vi "ReadSetPoint Example.vi"() -> ()   [LabVIEW 2019]
uses:
  BrooksDLL.dll
panel:
  out "Unit Comment (if Pressure)":string
  out "Unit Comment (if Flow)":string
  out "Unit Code":u8
  out "Set Point Value":sgl format="%.2f"
  out "S2 String":string
  out "S1 String":string
  out "S2":u8 format="%.0x"
  out "S1":u8 format="%.0x"
  out "Function Output Comment":string
  out "SetPoint %":sgl format="%.2f"
  out "output param":i32
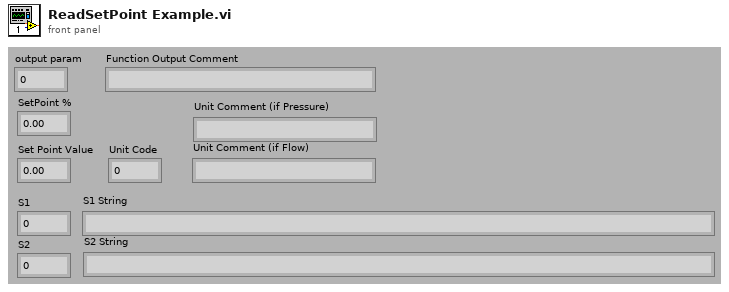
[diagram p1: front panel]
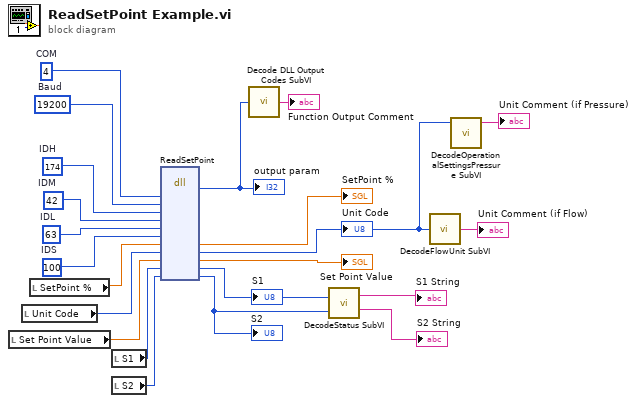
[diagram p0: block diagram]
diagram:
  w17 = u8 100  # IDS
  w18 = u8 63  # IDL
  w19 = u8 42  # IDM
  w20 = u8 174  # IDH
  w21 = 19200  # Baud
  w22 = 4  # COM
  n1 = local read "Set Point Value"() -> (w4:sgl)
  n2 = local read "Unit Code"() -> (w5:u8)
  n3 = local read "SetPoint %"() -> (w14:sgl)
  n4 = local read "S1"() -> (w9:u8)
  n5 = local read "S2"() -> (w10:u8)
  n6 = dll-call lib="G:/Developpement_de_Programmes/Programmes/Controle de pression/164J027_AD/Brooks DLL 1.0.1.0 32bit/Brooks DLL 1.0.1.0 Release 10032016/S Protocol/BrooksDLL.dll" fn="ReadSetPoint"("COM"=w22, "Baud"=w21, "IDH"=w20, "IDM"=w19, "IDL"=w18, "IDS"=w17, "SetPoint"=w14, "FlowUnit"=w5, "SetPointValue"=w4, "S1"=w9, "S2"=w10) -> (w16:i32, "SetPoint"=→"SetPoint %":sgl, "FlowUnit"=w2:u8, "SetPointValue"=→"Set Point Value":sgl, "S1"=w7:u8, "S2"=w8:u8)  [unwired: 9 in, 2 out]
  "output param" <- w16
  "S1" <- w7
  "S2" <- w8
  "Unit Code" <- w2
  n7 = call "Decode DLL Output Codes SubVI.vi"("Numeric"=w16) -> ("Function Output Comment"=→"Function Output Comment":string)
  n8 = call "DecodeStatus SubVI.vi"("S2"=w8, "S1"=w7) -> ("S2 String"=→"S2 String":string, "S1 String"=→"S1 String":string)
  n9 = call "DecodeFlowUnit SubVI.vi"("FlowUnit"=w2) -> ("Flow Unit Comment"=→"Unit Comment (if Flow)":string)
  n10 = call "DecodeOperationalSettingsPressure SubVI.vi"("PressureUnitCode"=w2) -> ("PressureUnitCode Comment"=→"Unit Comment (if Pressure)":string)  [unwired: 2 in, 2 out]
